vi "Write MetaData.vi"(8 "error in (no error)":errorcluster, 10 "MetaData":string, 11 "ExpData in":refnum<class "ExpData.lvclass">) -> (0 "error out":errorcluster, 3 "ExpData out":refnum<class "ExpData.lvclass">)   [LabVIEW 2015, in "ExpData.lvclass"]
uses:
  ExpData.lvclass
  ExpData.lvclass/ExpData.ctl
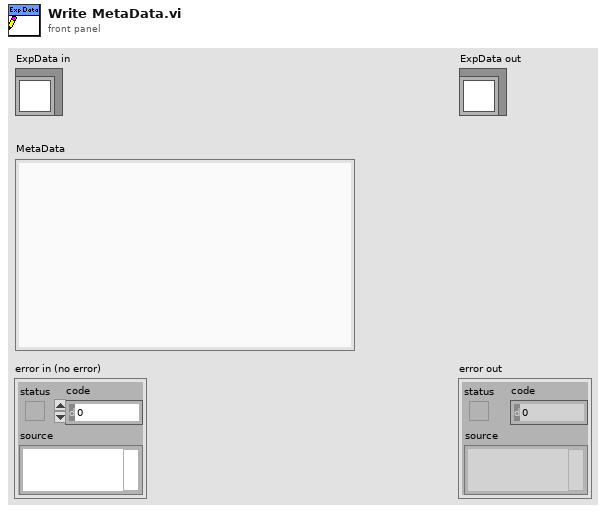
[diagram p1: front panel]
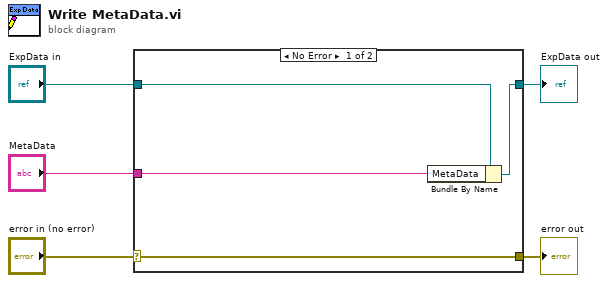
[diagram p0: block diagram]
diagram:
  n1 = case shown="No Error" "error in (no error)" {
    selector: "error in (no error)" -> [w9 w10]
    tunnel: [w9 w10] -> w4
    tunnel: [w7 w11] -> w2
    tunnel: "ExpData in" -> [w8 w11]
    tunnel: "MetaData" -> [w6 _]
    frame No Error {
      n2 = Bundle By Name(cluster=w8, "MetaData"=w6) -> (w7:refnum<class "ExpData.lvclass">)
    }
    frame Error {
    }
  }
  "error out" <- w4
  "ExpData out" <- w2
